vi "Actor Queue.vi"(6 "Creator":refnum<data-value>, 8 "Creator Alias":string, 9 "Self Alias":string, 10 "Queue of Queue Self":refnum<queue>, 11 "Queue jettl":refnum<class "Queue jettl.lvclass">) -> ()   [LabVIEW 2021, in "jettl.lvlib" / "Base Queue jettl.lvlib" / "Base Queue jettl.lvclass"]
uses:
  Base Queue jettl.lvclass
  Queue jettl/Queue jettl.lvclass
  C:/git/jettl/src/jettl/jettl/jettl.lvclass
  Msg Strategy/Msg Strategy.lvclass
  C:/git/jettl/src/jettl/Queue jettl/Queue jettl.lvclass
  jettl Msg Last Ack Queue/Last Ack Queue Msg Strategy/Last Ack Queue Msg Strategy.lvclass
  C:/git/jettl/src/jettl/Msg Strategy/Msg Strategy.lvclass
  Base Queue jettl.lvclass/Base Queue jettl.ctl
  Self Queue/Self Queue.lvlib
  jettl.lvlib
  Queue Mailbox/Queue Mailbox.lvlib
  jettl Msg Last Ack Queue/jettl Msg Last Ack Queue.lvlib
  C:/git/jettl/src/jettl Msg Merge Error/Merge Error/Merge Error.lvclass
  C:/git/jettl/src/jettl Msg Create Queue/Create Queue/Create Queue.lvclass
  C:/git/jettl/src/jettl Msg Create Event/Event Create/Create Event.lvclass
  C:/git/jettl/src/jettl Msg Override Error/Override Error/Override Error.lvclass
  C:/git/jettl/src/jettl Msg Setup/Setup/Setup.lvclass
  C:/git/jettl/src/jettl Msg Teardown/Teardown/Teardown.lvclass
  C:/git/jettl/src/jettl/jettl Msg Last Ack Event/Last Ack Event/Last Ack Event.lvclass
  C:/git/jettl/src/jettl/jettl Msg Last Ack Queue/Last Ack Queue/Last Ack Queue.lvclass
  C:/git/jettl/src/jettl/Base Queue jettl/Base Queue jettl/Base Queue jettl.lvclass
  C:/git/jettl/src/jettl/jettl Msg Last Ack Queue/Last Ack Queue Msg Strategy/Last Ack Queue Msg Strategy.lvclass
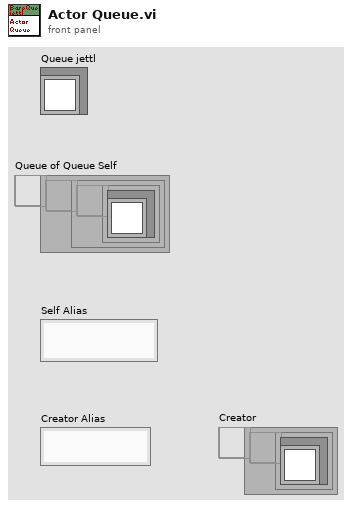
[diagram p1: front panel]
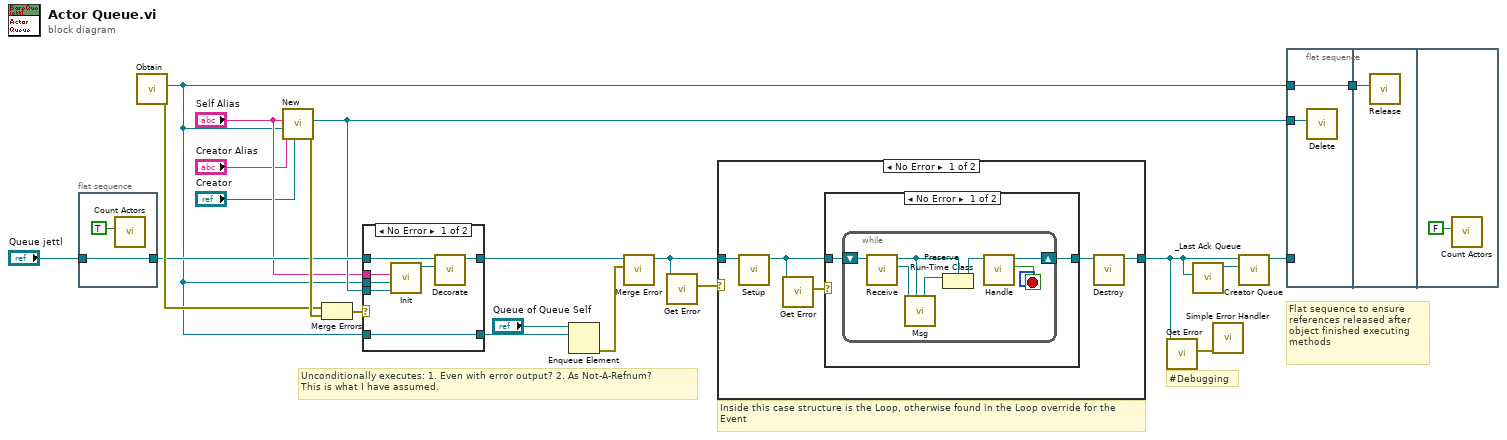
[diagram p0: block diagram]
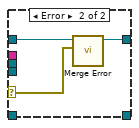
[diagram p2: hidden frame]
diagram:
  # "Inside this case structure is the Loop, otherwise found in the Loop override for the Event"
  # "Flat sequence to ensure references released after object finished executing methods"
  # "#Debugging"
  # "Unconditionally executes: 1. Even with error output? 2. As Not-A-Refnum?\nThis is what I have assumed."
  n1 = flat-sequence {
    tunnel: [w22] -> w11
    tunnel: "Queue jettl" -> [w22]
    frame #0 {
      n2 = call "Count Actors.vi"("Increment?"=TRUE) -> ()  [unwired: 11 in]
    }
  }
  n3 = call "Obtain.vi"() -> ("error out"=w12:errorcluster, "Self Queue"=w6:refnum<data-value>)  [unwired: 10 in]
  n4 = call "New.vi"("Creator Queue"="Creator", "Creator Queue Alias"="Creator Alias", "Self Queue"=w6, "Self Queue Alias"="Self Alias") -> ("error out"=w13:errorcluster, "Queue Mailbox"=w8:refnum<data-value>)  [unwired: 6 in]
  n5 = Merge Errors(w12, w13) -> (w14:errorcluster)
  n6 = case shown="No Error" w14 {
    selector: w14 -> [_ w32]
    tunnel: [w29 w33] -> w19
    tunnel: w11 -> [w30 w31]
    tunnel: w6 -> [w28 _]
    tunnel: [w28 _] -> w18
    tunnel: w8 -> [w26 _]
    tunnel: "Self Alias" -> [w25 _]
    tunnel: w6 -> [w24 _]
    frame No Error {
      n7 = call "Init.vi"("Queue Mailbox"=w26, "Queue Self"=w24, "Queue Self Alias"=w25) -> ("Base Queue jettl out"=w27:refnum<class "Base Queue jettl.lvclass">)  [unwired: 8 in]
      n8 = call-dynamic "Decorate.vi"("Queue jettl"=w27, "Queue jettl in"=w30) -> ("Queue jettl out"=w29:refnum<class "Queue jettl.lvclass">)  [unwired: 9 in]
    }
    frame Error {
      n9 = call-dynamic "Merge Error.vi"("Error"=w32, "Merge Error in"=w31) -> ("Merge Error out"=w33:refnum<class "Queue jettl.lvclass">)  [unwired: 9 in]
    }
  }
  n10 = Enqueue Element(queue="Queue of Queue Self", element=w18) -> (error out=w20:errorcluster)  [unwired: 2 in, 2 out]
  n11 = call-dynamic "Merge Error.vi"("Error"=w20, "Merge Error in"=w19) -> ("Merge Error out"=w21:refnum<class "Queue jettl.lvclass">)  [unwired: 9 in]
  n12 = call-dynamic "Get Error.vi"("jettl in"=w21) -> ("Error"=w17:errorcluster)  [unwired: 10 in]
  n13 = case shown="No Error" w17 {
    tunnel: w21 -> [w35 w49]
    tunnel: [w34 w49] -> w3
    frame No Error {
      n14 = call-dynamic "Setup.vi"("Setup in"=w35) -> ("Setup out"=w37:refnum<class "Queue jettl.lvclass">)  [unwired: 10 in]
      n15 = call-dynamic "Get Error.vi"("jettl in"=w37) -> ("Error"=w38:errorcluster)  [unwired: 10 in]
      n16 = case shown="No Error" w38 {
        tunnel: [w40 w48] -> w36
        tunnel: w37 -> [w39 w48]
        frame No Error {
          n17 = while "Queue Loop" {
            shift-right: [w47] -> w40
            shift-left: w39 -> [w46]
            stop <- w44 stop-if-true
            n18 = call-dynamic "Receive.vi"("Queue jettl in"=w46) -> ("Msg Strategy"=w45:refnum<class "Msg Strategy.lvclass">, "Queue jettl out"=w43:refnum<class "Queue jettl.lvclass">)  [unwired: 9 in]
            n19 = call-dynamic "Msg.vi"("jettl in"=w43, "Msg Strategy in"=w45) -> ("jettl out"=w41:refnum<class "jettl.lvclass">)  [unwired: 9 in]
            n20 = Preserve Run-Time Class(object in=w41, 2:w43) -> (object out=w42:refnum<class "Queue jettl.lvclass">)  [unwired: 1 in, 1 out]
            n21 = call-dynamic "Handle.vi"("jettl in"=w42) -> ("Destroy?"=w44:bool, "jettl out"=w47:refnum<class "Queue jettl.lvclass">)  [unwired: 9 in]
          }
        }
        frame Error {
        }
      }
      n22 = call-dynamic "Destroy.vi"("jettl in"=w36) -> ("jettl out"=w34:refnum<class "Queue jettl.lvclass">)  [unwired: 10 in]
    }
    frame Error {
    }
  }
  n23 = call-dynamic "Get Error.vi"("jettl in"=w3) -> ("Error"=w9:errorcluster)  [unwired: 10 in]
  n24 = call "_Last Ack Queue.vi"("Queue jettl"=w3) -> ("Last Ack Queue Msg Strategy out"=w1:refnum<class "Last Ack Queue Msg Strategy.lvclass">)  [unwired: 10 in]
  n25 = call <vilib>:"Simple Error Handler.vi"("error in (no error)"=w9) -> ()  [unwired: 4 in, 5 out]
  n26 = call-dynamic "Creator Queue.vi"("Msg Strategy"=w1, "Queue jettl in"=w3) -> ("Queue jettl out"=w2:refnum<class "Queue jettl.lvclass">)  [unwired: 9 in]
  n27 = flat-sequence {
    tunnel: w8 -> [w51]
    tunnel: [w50] -> w10
    tunnel: w6 -> [w50]
    tunnel: w2 -> [_]
    tunnel: w10 -> [w52]
    frame #0 {
      n28 = call "Delete.vi"("Queue Mailbox"=w51) -> ()  [unwired: 10 in, 1 out]
    }
    frame #1 {
      n29 = call "Release.vi"("Self Queue"=w52) -> ()  [unwired: 10 in, 1 out]
    }
    frame #2 {
      n30 = call "Count Actors.vi"("Increment?"=FALSE) -> ()  [unwired: 11 in]
    }
  }
